vi "To Instrument Session Init and Close Behavior.vi"(10 "session exists":bool, 11 "initialize and close session behavior":T2) -> (3 "instrument initialize and close session behavior":T1)   [LabVIEW 2020, in "MeasurementLink Session Management.lvlib" / "Session Reservation.lvclass"]
uses:
  Session Reservation.lvclass
  Session Reservation.lvclass/Session Reservation.ctl
  MeasurementLink Instrument/IInstrument/Initialize and Close Session Behavior.ctl
  MeasurementLink Instrument/IInstrument/IInstrument.lvclass
  Initialize and Close Session Behavior.ctl
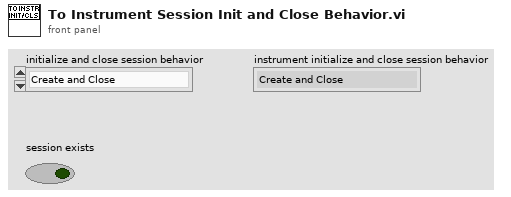
[diagram p1: front panel]
types:
  T1 = typedef "MeasurementLink Instrument.lvlib/IInstrument.lvclass/Initialize and Close Session Behavior.ctl" = enum16{"Create and Close", "Attach and Detach", "Create and Detach", "Attach and Close"}
  T2 = typedef "MeasurementLink Session Management.lvlib/Session Reservation.lvclass/Initialize and Close Session Behavior.ctl" = enum16{"Create and Close", "Attach and Detach", "Create and Detach", "Attach and Close", "Auto"}
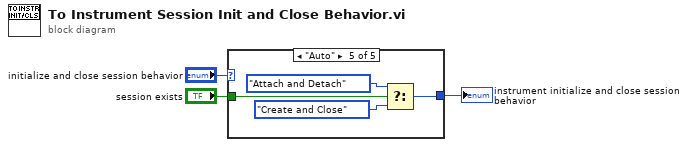
[diagram p0: block diagram]
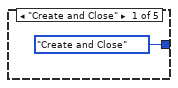
[diagram p2: hidden frame]
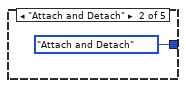
[diagram p3: hidden frame]
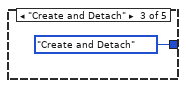
[diagram p4: hidden frame]
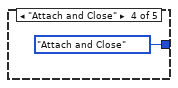
[diagram p5: hidden frame]
diagram:
  n1 = case shown="\"Auto\"" "initialize and close session behavior" {
    tunnel: [Initialize_and_Close_Session_Behavior."Create and Close" ("instrument initialize and close session behavior") Initialize_and_Close_Session_Behavior."Attach and Detach" ("instrument initialize and close session behavior") Initialize_and_Close_Session_Behavior."Create and Detach" ("instrument initialize and close session behavior") Initialize_and_Close_Session_Behavior."Attach and Close" ("instrument initialize and close session behavior") w8] -> w2
    tunnel: "session exists" -> [_ _ _ _ w11]
    frame "Create and Close" {
    }
    frame "Attach and Detach" {
    }
    frame "Create and Detach" {
    }
    frame "Attach and Close" {
    }
    frame "Auto" {
      n2 = Select(t=Initialize_and_Close_Session_Behavior."Attach and Detach" ("instrument initialize and close session behavior"), s=w11, f=Initialize_and_Close_Session_Behavior."Create and Close") -> (s? t:f=w8:T1)
    }
  }
  "instrument initialize and close session behavior" <- w2
